vi "CliGetCpInfo.vi"(0 "ref in":u64, 11 "error in (no error)":errorcluster) -> (2 "Max PDULength":i32, 3 "Max Connections":i32, 4 "ref out":u64, 6 "Result":i32, 13 "MaxBus Rate":i32, 14 "Max MPI Rate":i32, 15 "error out":errorcluster)   [LabVIEW 2020, in "Snap7.lvlib"]
uses:
  Snap7.lvlib
  windows/lv_snap7.dll
panel:
  in  "var_Info":T1
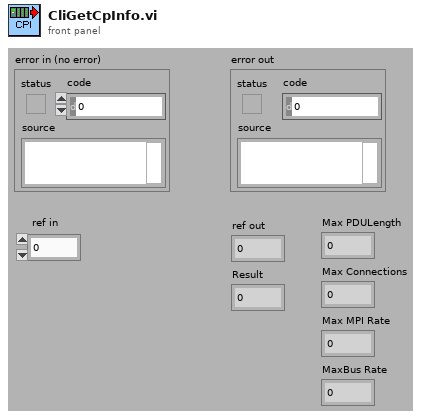
[diagram p1: front panel]
types:
  T1 = cluster{"Max PDULength var":i32, "Max Connections var":i32, "Max MPI Rate var":i32, "MaxBus Rate var":i32}
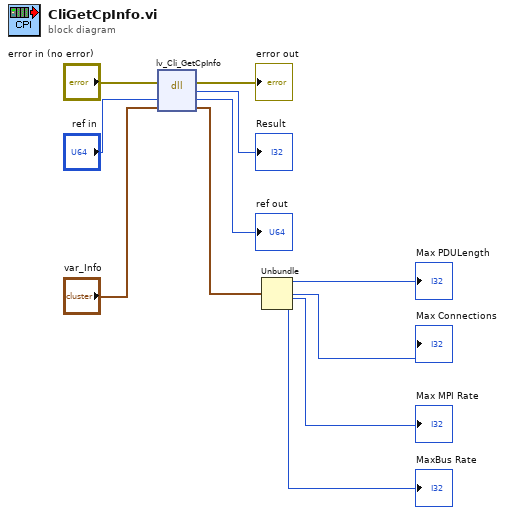
[diagram p0: block diagram]
diagram:
  n1 = dll-call lib="PTH2iabs CUsersFeng项目HLCEPS300-1老性能试验台SourcesSnap7libwindowslv_snap7.dll" fn="lv_Cli_GetCpInfo"(error in="error in (no error)", "Client"="ref in", "var_Info"="var_Info") -> (error out=→"error out":errorcluster, "return type"=→"Result":i32, "Client"=→"ref out":u64, "var_Info"=w6:T1)  [unwired: 2 in, 1 out]
  n2 = Unbundle(w6) -> ("Max PDULength var"=→"Max PDULength":i32, "Max Connections var"=→"Max Connections":i32, "Max MPI Rate var"=→"Max MPI Rate":i32, "MaxBus Rate var"=→"MaxBus Rate":i32)
